vi "Host_PhotonCounter_tester2.vi"() -> ()   [LabVIEW 2012]
uses:
  <vilib>/FPGAPlugInAG/PXIe-7962R/niLvFpga_Open_PXIe-7962R.vi
  <vilib>/rvi/interface/common/dynamic/niFpgaDynamicAddResources.vi
  <vilib>/FPGAPlugInAG/Dynamic/niLvFpga_Reset_Dynamic.vi
  <vilib>/Utility/error.llb/Error Cluster From Error Code.vi
  <vilib>/rvi/errors/niLvFpgaAdjustHostInterfaceError.vi
  <vilib>/FPGAPlugInAG/Dynamic/niLvFpga_Close_Dynamic.vi
  <vilib>/rvi/interface/nirviOpenFPGA/nirviOpenFPGA.xnode
  FPGA Bitfiles/PhotonCounter_tester2.lvbitx
  <vilib>/rvi/interface/nirviMethod/nirviMethod.xnode
  <vilib>/rvi/interface/nirviReadWriteControl/nirviReadWriteControl.xnode
  <vilib>/rvi/interface/nirviCloseFPGA/nirviCloseFPGA.xnode
  <vilib>/rvi/interface/Simulation/niFpgaSimulationCallBeginRW.vi
  NiFpgaLv.dll
  <vilib>/FPGAPlugInAG/Dynamic/niLvFpga_ReadFifo_Dynamic.vi
  <vilib>/rvi/errors/niLvFpgaMergeErrorWithErrorCode.vi
panel:
  out "Timeout counter 2":u64
  out "Sample counter 2":u64
  out "Timeout counter":u64
  out "Sample counter Acq":u64
  out "Sample counter":u64
  out "Laser pulses per pixel":dbl
  in  "Laser pulse frequency":dbl=80000000.0 format="%#_6p"
  out "Pixel time":dbl
  out "Interloop FIFO overflow":bool
  out "ToHost FIFO Overflow":bool
  out "Interloop FIFO timeout":bool
  in  "Reset":bool
  in  "Quit":bool
  out "Sampling frequency":dbl format="%#_6p"
  out "Sampling interval":dbl format="%#_6p"
  in  "Onboard clock frequency":dbl=500000000.0 format="%#_6p"
  # "Configuration"
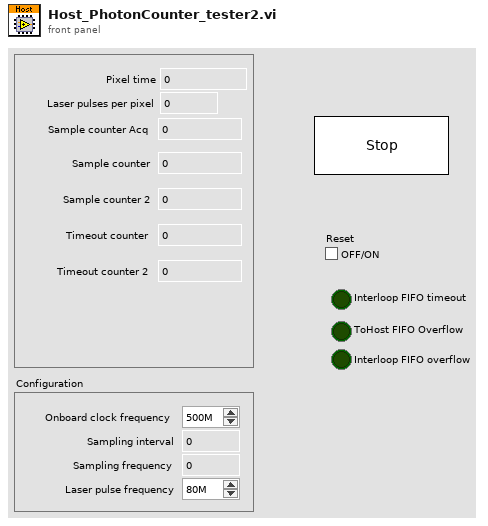
[diagram p1: front panel]
types:
  T1 = enum8{"Enabled", "Disabled", "Disabled and Grayed Out"}
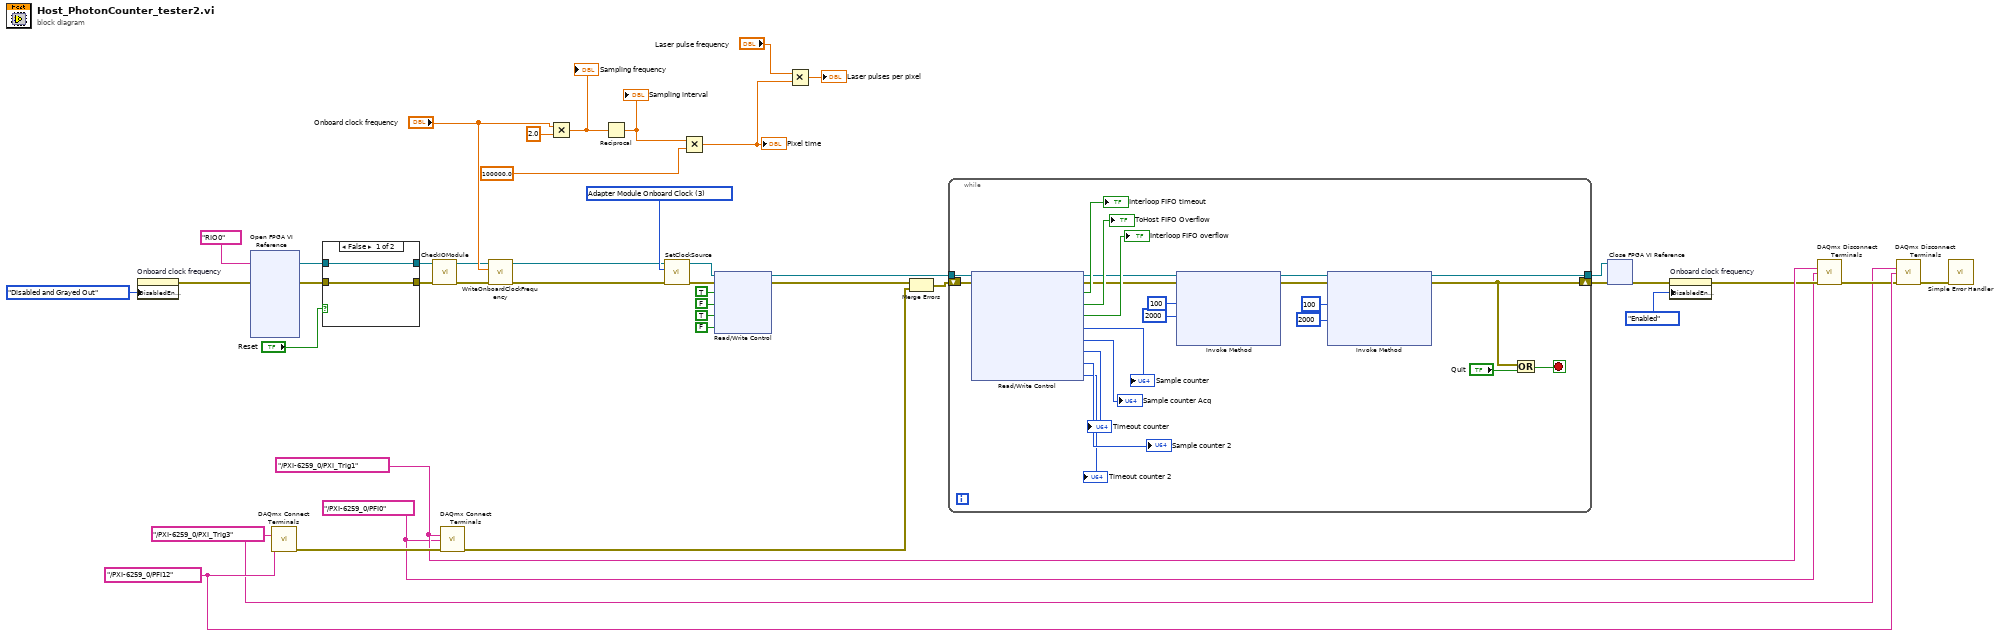
[diagram p0: block diagram]
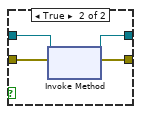
[diagram p2: hidden frame]
diagram:
  w6 = tag "/PXI-6259_0/PFI0" ("destination terminal")
  w11 = tag "/PXI-6259_0/PXI_Trig1" ("source terminal")
  w14 = tag "/PXI-6259_0/PFI12" ("destination terminal")
  w7 = tag "/PXI-6259_0/PXI_Trig3" ("source terminal")
  w43 = u8 3 items=["Tristate"=0, "Sync Clock (PXIe only)"=2, "Adapter Module Onboard Clock"=3, "Strobe from Crosspoint Switch"=4, "Strobe Bypass"=5] ("Clock Source")
  n1 = property on="Onboard clock frequency" class="DigNum (strict)"("DisabledEnum"=T1."Disabled and Grayed Out" ("Disabled")) -> (error out=w32:errorcluster)  [unwired: 2 in, 1 out]
  n2 = xnode "Open FPGA VI Reference"("error in"=w32, "resource name"=tag "RIO0") -> ("FPGA VI Reference Out"=w23:refnum<k20>, "error out"=w21:errorcluster)
  n3 = call <vilib>:"DAQmx Connect Terminals.vi"("source terminal"=w7, "destination terminal"=w14) -> ("error out"=w13:errorcluster)  [unwired: 13 in]
  n4 = case shown="False" "Reset" {
    tunnel: w23 -> [w44 w49]
    tunnel: [w44 w48] -> w22
    tunnel: w21 -> [w45 w47]
    tunnel: [w45 w46] -> w20
    frame False {
    }
    frame True {
      n5 = xnode "Invoke Method"("FPGA VI Reference In"=w49, "error in"=w47) -> ("FPGA VI Reference Out"=w48:refnum<k20>, "error out"=w46:errorcluster)
    }
  }
  n6 = call "CheckIOModule.vi"("error in (no error)"=w20, "FPGA VI Reference In"=w22) -> ("error out"=w36:errorcluster, "FPGA VI Reference Out"=w28:refnum<k20>)  [unwired: 8 in]
  n7 = call <vilib>:"DAQmx Connect Terminals.vi"("source terminal"=w11, "destination terminal"=w6, "error in"=w13) -> ("error out"=w12:errorcluster)  [unwired: 12 in]
  n8 = call "WriteOnboardClockFrequency.vi"("error in (no error)"=w36, "Onboard clock frequency"="Onboard clock frequency", "FPGA VI Reference In"=w28) -> ("error out"=w4:errorcluster, "FPGA VI Reference Out"=w3:refnum<k20>)  [unwired: 7 in]
  n9 = Multiply(x="Onboard clock frequency", y=2.0) -> (x*y=w33:dbl)
  "Sampling frequency" <- w33
  n10 = Reciprocal(x=w33) -> (1/x=w25:dbl)
  "Sampling interval" <- w25
  n11 = call "SetClockSource.vi"("error in (no error)"=w4, "Clock Source"=w43, "FPGA VI Reference In"=w3) -> ("error out"=w41:errorcluster, "FPGA VI Reference Out"=w42:refnum<k20>)  [unwired: 7 in]
  n12 = Multiply(x=w25, y=100000.0) -> (x*y=w17:dbl)
  "Pixel time" <- w17
  n13 = xnode "Read/Write Control"("FPGA VI Reference In"=w42, "error in"=w41, "Commit"=TRUE, "Acq_Reset"=FALSE, "Acq_Reset"=TRUE, "Acq_Reset"=FALSE) -> ("FPGA VI Reference Out"=w1:refnum<k20>, "error out"=w2:errorcluster)
  n14 = Multiply(x="Laser pulse frequency", y=w17) -> (x*y=→"Laser pulses per pixel":dbl)
  n15 = Merge Errors(w2, w12) -> (w15:errorcluster)
  n16 = while {
    shift-right: [w52] -> w27
    shift-left: w15 -> [w69]
    tunnel: [w53] -> w26
    tunnel: w1 -> [w60]
    stop <- w70 stop-if-true
    n17 = xnode "Read/Write Control"("FPGA VI Reference In"=w60, "error in"=w69) -> ("FPGA VI Reference Out"=w65:refnum<k20>, "error out"=w64:errorcluster, "Interloop FIFO timeout"=→"Interloop FIFO timeout":bool, "ToHost FIFO Overflow"=→"ToHost FIFO Overflow":bool, "Interloop FIFO overflow"=→"Interloop FIFO overflow":bool, "Sample counter 1"=→"Sample counter":u64, "Sample counter Acq"=→"Sample counter Acq":u64, "Timeout counter 1"=→"Timeout counter":u64, "Sample counter 2"=→"Sample counter 2":u64, "Timeout counter 2"=→"Timeout counter 2":u64)
    n18 = xnode "Invoke Method"("FPGA VI Reference In"=w65, "error in"=w64, "Number of Elements"=u32 100, "Timeout (ms)"=2000) -> ("FPGA VI Reference Out"=w55:refnum<k20>, "error out"=w54:errorcluster)  [unwired: 2 out]
    n19 = xnode "Invoke Method"("FPGA VI Reference In"=w55, "error in"=w54, "Number of Elements"=u32 100, "Timeout (ms)"=2000) -> ("FPGA VI Reference Out"=w53:refnum<k20>, "error out"=w52:errorcluster)  [unwired: 2 out]
    n20 = Or(x=w52, y="Quit") -> (x .or. y?=w70:bool)
  }
  n21 = xnode "Close FPGA VI Reference"("FPGA VI Reference In"=w26, "error in"=w27) -> ("error out"=w30:errorcluster)
  n22 = property on="Onboard clock frequency" class="DigNum (strict)"(error in=w30, "DisabledEnum"=T1."Enabled" ("Disabled")) -> (error out=w10:errorcluster)  [unwired: 1 in, 1 out]
  n23 = call <vilib>:"DAQmx Disconnect Terminals.vi"("source terminal"=w11, "destination terminal"=w6, "error in"=w10) -> ("error out"=w9:errorcluster)  [unwired: 12 in]
  n24 = call <vilib>:"DAQmx Disconnect Terminals.vi"("source terminal"=w7, "destination terminal"=w14, "error in"=w9) -> ("error out"=w8:errorcluster)  [unwired: 12 in]
  n25 = call <vilib>:"Simple Error Handler.vi"("error in (no error)"=w8) -> ()  [unwired: 4 in, 5 out]
